vi "checkFinishPreparePenaltyEnemyPlay.vi"(8 "error in (no error)":errorcluster, 10 "Game":refnum<class "Game.lvclass">, 11 "PreparePenaltyEnemyPlay in":refnum<class "PreparePenaltyEnemyPlay.lvclass">) -> (0 "error out":errorcluster, 2 "Boolean":bool, 3 "PreparePenaltyEnemyPlay out":refnum<class "PreparePenaltyEnemyPlay.lvclass">)   [LabVIEW 2018, in "PreparePenaltyEnemyPlay.lvclass"]
uses:
  PreparePenaltyEnemyPlay.lvclass
  Game_class/Game.lvclass
  Referee_class/command_interpreted.ctl
  Game_class/Game.lvclass/Game.ctl
  Referee_class/Referee.lvclass/Referee.ctl
  Events_class/Events.lvclass/Events.ctl
  Game_class/Read Referee.vi
  Game_class/Read EventsRef.vi
  Events_class/Read ball_out.vi
  Events_class/Read touch.vi
  Events_class/Read id_touch.vi
  Referee_class/Read command_interpreted.vi
  Referee_class/Referee.lvclass
  Events_class/Events.lvclass
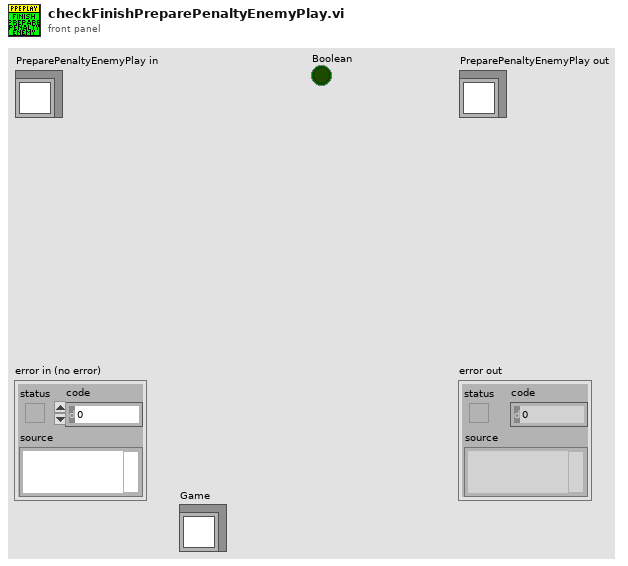
[diagram p1: front panel]
types:
  T1 = typedef "command_interpreted.ctl" = enum16{"Goal Ally", "Goal Enemy", "Ball Placement Enemy", "Ball Placement Ally", "Normal Half Time", "Extra Time  Break", "Extra Half Time", "None", "Post Game", "PKA Normal Start", "Prepare Kickoff Ally", "PKE Normal Start", "Prepare Kickoff Enemy", "Force Start", "Halt", "Timeout", "Prepare Penalty Ally", "Prepare Penalty Enemy", "PPA NormalStart", "PPE Normal Start", "Indirect Free Ally", "Direct Free Enemy", "Direct Free Ally", "Indirect Free Enemy", "Stop"}
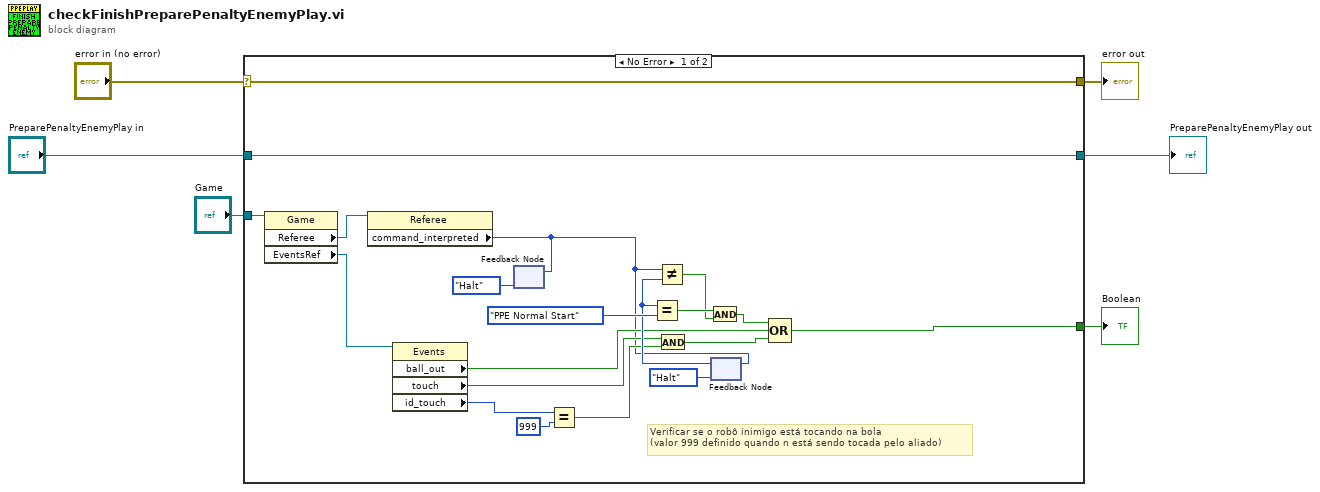
[diagram p0: block diagram]
diagram:
  n1 = case shown="No Error" "error in (no error)" {
    selector: "error in (no error)" -> [w25 w28]
    tunnel: [w25 w28] -> w5
    tunnel: [w26 w27] -> w3
    tunnel: "PreparePenaltyEnemyPlay in" -> [w26 w27]
    tunnel: "Game" -> [w19 _]
    tunnel: [w15 _] -> w1
    frame No Error {
      # "Verificar se o robô inimigo está tocando na bola\n(valor 999 definido quando n está sendo tocada pelo aliado)"
      n2 = property class="Game"(reference=w19) -> ("Referee"=w24:refnum<class "Referee.lvclass">, "EventsRef"=w18:refnum<class "Events.lvclass">)  [unwired: 1 in, 2 out]
      n3 = property class="Referee"(reference=w24) -> ("command_interpreted"=w9:T1)  [unwired: 1 in, 2 out]
      n4 = property class="Events"(reference=w18) -> ("ball_out"=w16:bool, "touch"=w12:bool, "id_touch"=w14:i32)  [unwired: 1 in, 2 out]
      n5 = feedback #1(command_interpreted."Halt" ("command_interpreted")) -> ()  [unwired: 1 in]
      n6 = feedback-in #1(w9) -> ()
      n7 = Equal?(x=w14, y=999) -> (x = y?=w11:bool)
      n8 = And(x=w12, y=w11) -> (x .and. y?=w10:bool)
      n9 = feedback #2(command_interpreted."Halt" ("command_interpreted")) -> (w21:T1)
      n10 = Equal?(x=w21, y=command_interpreted."PPE Normal Start" ("command_interpreted")) -> (x = y?=w22:bool)
      n11 = Not Equal?(x=w9, y=w21) -> (x != y?=w8:bool)
      n12 = And(x=w22, y=w8) -> (x .and. y?=w17:bool)
      n13 = feedback-in #2(w9) -> ()
      n14 = Compound Arithmetic op=OR(w17, w16, w10) -> (w15:bool)
    }
    frame Error {
    }
  }
  "error out" <- w5
  "PreparePenaltyEnemyPlay out" <- w3
  "Boolean" <- w1
